vi "PM100-Get Power Ranges.vi"(0 "VISA Refnum in":refnum<visa-resource-name>, 11 "error in (no error)":errorcluster) -> (4 "VISA Refnum out":refnum<visa-resource-name>, 8 "Ranges":string[](array[string]), 15 "error out":errorcluster)   [LabVIEW 2015]
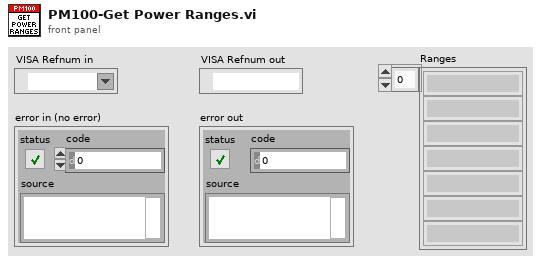
[diagram p1: front panel]
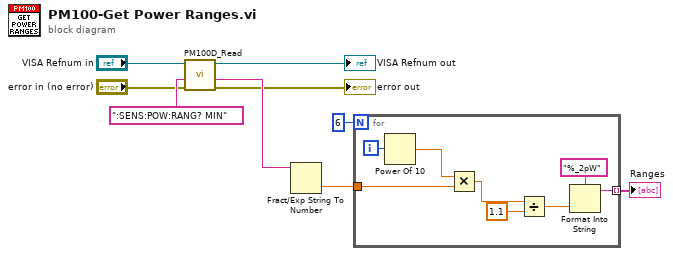
[diagram p0: block diagram]
diagram:
  n1 = call "PM100D_Read.vi"("error in (no error)"="error in (no error)", "Command"=":SENS:POW:RANG? MIN", "VISA in"="VISA Refnum in") -> ("error out"=→"error out":errorcluster, "ReadValue"=w6:string, "VISA out"=→"VISA Refnum out":refnum<visa-resource-name>)  [unwired: 6 in]
  n2 = Fract/Exp String To Number(string=w6) -> (number=w3:dbl)  [unwired: 3 in, 1 out]
  n3 = for {
    N: 6 -> [_]
    tunnel: w3 -> [w13]
    tunnel: [w10] -> w2 mode=indexing
    i -> [w12]
    n4 = Power Of 10(x=w12) -> (10^x=w11:dbl)
    n5 = Multiply(x=w11, y=w13) -> (x*y=w17:dbl)
    n6 = Divide(x=w17, y=1.1) -> (x/y=w15:dbl)
    n7 = Format Into String(format string="%_2pW", w15) -> (resulting string=w10:string)  [unwired: 2 in, 1 out]
  }
  "Ranges" <- w2
